vi "ActionVIOnLoad.vi"(8 "error in (no error)":errorcluster, 11 "Device Item Ref in":T1 format="%.0x") -> (0 "error out":errorcluster, 3 "Device Item Ref out":T1 format="%.0x")   [LabVIEW 2019, in "Protection and Counter Addon System Explorer.lvlib"]
uses:
  Protection and Counter Addon System Explorer.lvlib
  <vilib>/NI VeriStand/Custom Device API/Custom Device Item Ref.ctl
  NationalInstruments.VeriStand.SystemDefinitionAPI
  Shared/SubVIs/GUID Lookup.vi
  <vilib>/NI VeriStand/Custom Device Tools/Custom Device Utility Library/NI VeriStand - Search for Item by GUID.vi
  <vilib>/NI VeriStand/Custom Device API/Custom Device API.lvlib
  Shared/Protection and Counter Addon Shared.lvlib
  <vilib>/NI VeriStand/Custom Device Tools/Custom Device Utility Library/Custom Device Utility Library.lvlib
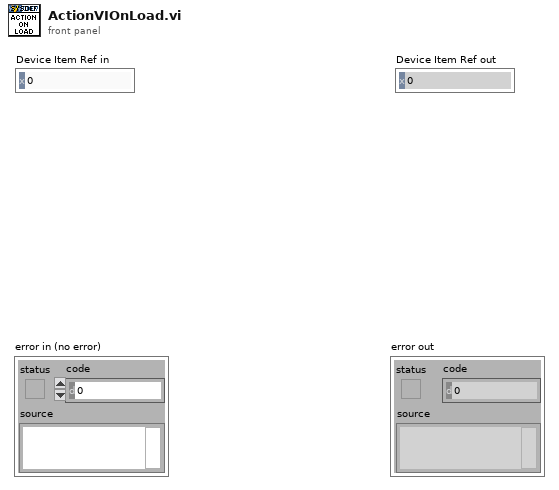
[diagram p1: front panel]
types:
  T1 = typedef "Custom Device API.lvlib/Custom Device Item Ref.ctl" = u64
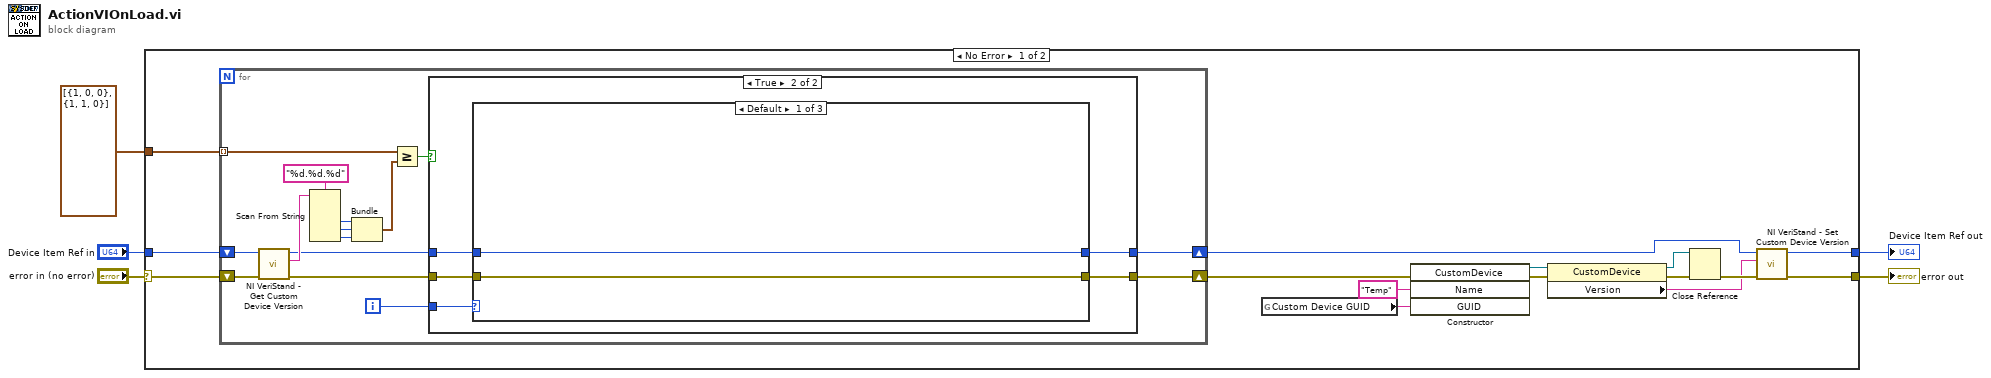
[diagram p0: block diagram]
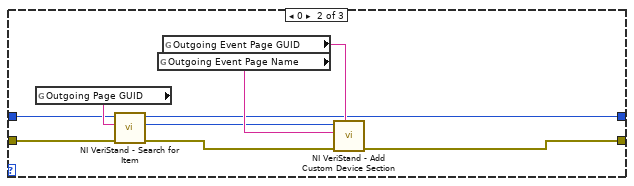
[diagram p3: hidden frame]
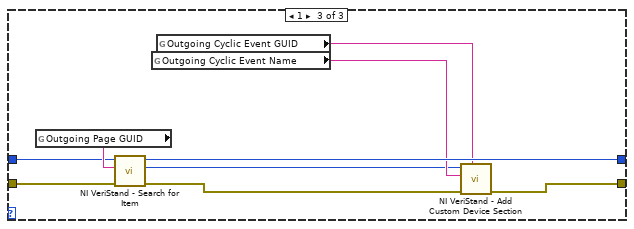
[diagram p4: hidden frame]
diagram:
  n1 = case shown="No Error" "error in (no error)" {
    selector: "error in (no error)" -> [w13 w64]
    tunnel: [w8 w64] -> w4
    tunnel: "Device Item Ref in" -> [w12 w63]
    tunnel: [w6 w63] -> w2
    tunnel: cluster{i32, i32, i32}[] [{1, 0, 0}, {1, 1, 0}] -> [w10 _]
    frame No Error {
      n2 = for {
        tunnel: w10 -> [w28] mode=indexing
        shift-right: [w23] -> w9
        shift-left: w13 -> [w30]
        shift-right: [w22] -> w11
        shift-left: w12 -> [w29]
        i -> [w21]
        n3 = call <vilib>:"NI VeriStand - Get Custom Device Version.vi"("error in (no error)"=w30, "Device Ref in"=w29) -> ("error out"=w25:errorcluster, "Value"=w33:string, "Device Ref out"=w24:T1)  [unwired: 7 in]
        n4 = Scan From String(format string="%d.%d.%d", input string=w33) -> (output 1=w34:i32, output 2=w35:i32, output 3=w31:i32)  [unwired: 5 in, 3 out]
        n5 = Bundle(w34, w35, w31) -> (w27:cluster{i32, i32, i32})  [unwired: 1 in]
        n6 = Greater Or Equal?(x=w28, y=w27) -> (x >= y?=w26:bool)
        n7 = case shown="True" w26 {
          tunnel: w25 -> [w37 w42]
          tunnel: w24 -> [w36 w41]
          tunnel: [w37 w39] -> w23
          tunnel: [w36 w40] -> w22
          tunnel: w21 -> [_ w38]
          frame False {
          }
          frame True {
            n8 = case shown="Default" w38 {
              tunnel: w42 -> [w43 w50 w61]
              tunnel: w41 -> [w44 w49 w60]
              tunnel: [w44 w46 w59] -> w40
              tunnel: [w43 w45 w56] -> w39
              frame Default {
              }
              frame 0 {
                n9 = global read "GUID Lookup.vi" "Outgoing Page GUID"() -> (w51:string)
                n10 = call-poly <vilib>:"NI VeriStand - Search for Item.vi"("error in"=w50, "Item GUID"=w51, "Section Ref in"=w49) -> ("error out"=w48:errorcluster, "Item Ref"=w47:T1, "Section Ref out"=w46:T1)  [unwired: 5 in, 1 out]
                n11 = global read "GUID Lookup.vi" "Outgoing Event Page Name"() -> (w53:string)
                n12 = global read "GUID Lookup.vi" "Outgoing Event Page GUID"() -> (w52:string)
                n13 = call <vilib>:"NI VeriStand - Add Custom Device Section.vi"("GUID (Default Section)"=w52, "error in (no error)"=w48, "Section Name"=w53, "Parent Ref in"=w47) -> ("error out"=w45:errorcluster)  [unwired: 4 in, 3 out]
              }
              frame 1 {
                n14 = global read "GUID Lookup.vi" "Outgoing Page GUID"() -> (w62:string)
                n15 = call-poly <vilib>:"NI VeriStand - Search for Item.vi"("error in"=w61, "Item GUID"=w62, "Section Ref in"=w60) -> ("error out"=w55:errorcluster, "Item Ref"=w54:T1, "Section Ref out"=w59:T1)  [unwired: 5 in, 1 out]
                n16 = global read "GUID Lookup.vi" "Outgoing Cyclic Event Name"() -> (w58:string)
                n17 = global read "GUID Lookup.vi" "Outgoing Cyclic Event GUID"() -> (w57:string)
                n18 = call <vilib>:"NI VeriStand - Add Custom Device Section.vi"("GUID (Default Section)"=w57, "error in (no error)"=w55, "Section Name"=w58, "Parent Ref in"=w54) -> ("error out"=w56:errorcluster)  [unwired: 4 in, 3 out]
              }
            }
          }
        }
      }
      n19 = global read "GUID Lookup.vi" "Custom Device GUID"() -> (w7:string)
      n20 = constructor class="CustomDevice"(error in=w9, "Name"="Temp", "GUID"=w7) -> (reference out=w20:refnum<k24>, error out=w19:errorcluster)  [unwired: 2 in, 3 out]
      n21 = property class="CustomDevice"(reference=w20, error in=w19) -> (reference out=w17:refnum<k24>, error out=w18:errorcluster, "Version"=w15:string)
      n22 = Close Reference(reference=w17, error in (no error)=w18) -> (error out=w16:errorcluster)
      n23 = call <vilib>:"NI VeriStand - Set Custom Device Version.vi"("error in (no error)"=w16, "Value"=w15, "Device Ref in"=w11) -> ("error out"=w8:errorcluster, "Device Ref out"=w6:T1)  [unwired: 7 in]
    }
    frame Error {
    }
  }
  "error out" <- w4
  "Device Item Ref out" <- w2
